vi "GetHelp.vi"(11 "SetConditionalSymbol in":refnum<class "SetConditionalSymbol.lvclass">) -> (2 "Help":string, 3 "SetConditionalSymbol out":refnum<class "SetConditionalSymbol.lvclass">)   [LabVIEW 2014, in "SetConditionalSymbol.lvclass"]
uses:
  SetConditionalSymbol.lvclass
panel:
  in  "HelpText":string="LabVIEWCLI -OperationName SetConditionalSymbol -ProjectPath <path of LabVIEW project>  -Symbol <name of the symbol in the project>  -Value <value the symbol should be set to>\n\n -ProjectPath : Specifies the full path to the LabVIEW project (.lvproj) file that contains the conditional symbol. \n -Symbol : Specifies the name of the conditional symbol. \n -Value : Specifies the string value of the conditional symbol.\n"
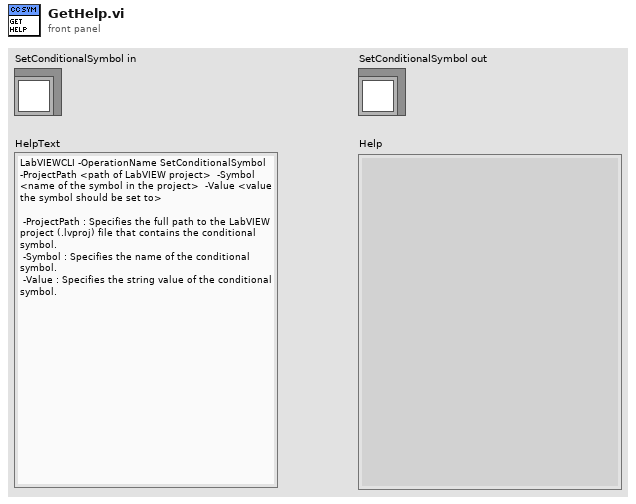
[diagram p1: front panel]
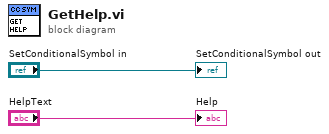
[diagram p0: block diagram]
diagram:
  "SetConditionalSymbol out" <- "SetConditionalSymbol in"
  "Help" <- "HelpText"
